vi "Set_RegDest.vi"(8 "error in (no error)":errorcluster, 10 "data":T1, 11 "Class in":refnum<class "IB_RegDest.lvclass">) -> (0 "error out":errorcluster, 3 "Class out":refnum<class "IB_RegDest.lvclass">)   [LabVIEW 2020, in "IB_RegDest.lvclass"]
uses:
  <vilib>/AppBuilder/IB_Classes/RegDest/IB_RegDest.lvclass
  <vilib>/AppBuilder/IB_Classes/RegDest/IB_RegDest.lvclass/IB_RegDest.ctl
  <vilib>/AppBuilder/IB_Classes/RegDest/IB_RegDest.ctl
  <vilib>/AppBuilder/IB_Classes/RegData/IB_RegData.lvclass
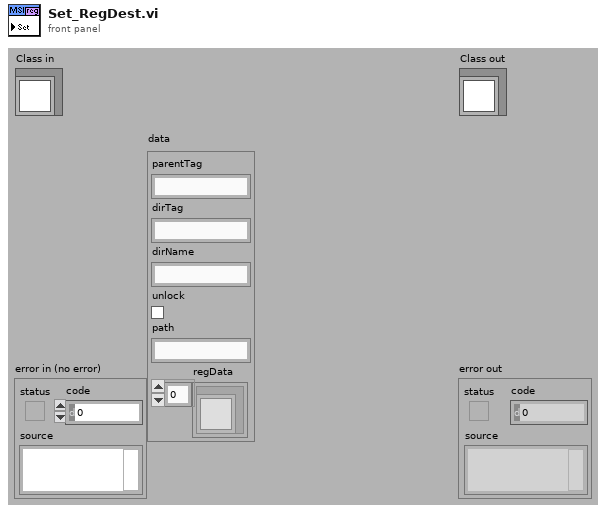
[diagram p1: front panel]
types:
  T1 = typedef "IB_RegDest.ctl" = cluster{"parentTag":string, "dirTag":string, "dirName":string, "unlock":bool, "path":string, "regData":refnum<class "IB_RegData.lvclass">[]}
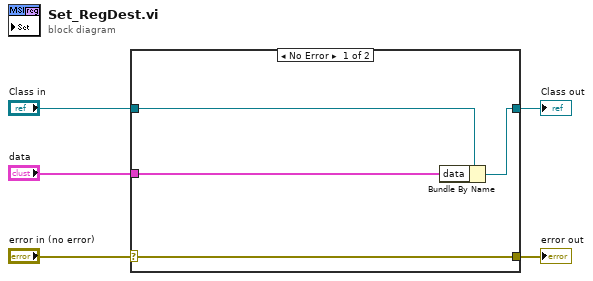
[diagram p0: block diagram]
diagram:
  n1 = case shown="No Error" "error in (no error)" {
    selector: "error in (no error)" -> [w9 w10]
    tunnel: [w9 w10] -> w4
    tunnel: [w7 w11] -> w2
    tunnel: "Class in" -> [w8 w11]
    tunnel: "data" -> [w6 _]
    frame No Error {
      n2 = Bundle By Name(cluster=w8, "data"=w6) -> (w7:refnum<class "IB_RegDest.lvclass">)
    }
    frame Error {
    }
  }
  "error out" <- w4
  "Class out" <- w2
